vi "CRYGet detailed path information.vi"(11 "complete path":path) -> (2 "portion type":i16, 3 "longest valid portion":path)   [LabVIEW 2013]
panel:
  out "stripped?":bool
  # "0: empty\n1: directory\n2: existing file\n3: valid new file\n4: Not a Path"
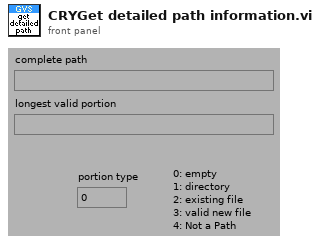
[diagram p1: front panel]
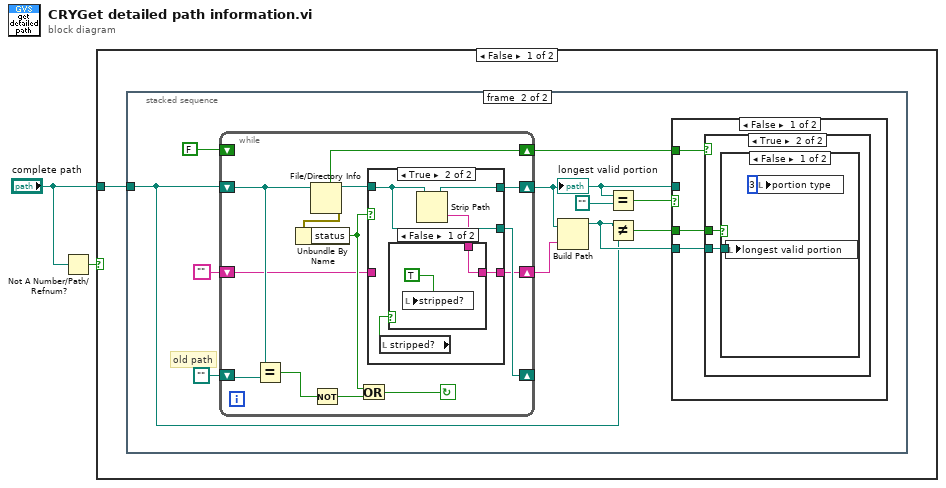
[diagram p0: block diagram]
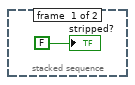
[diagram p2: hidden frame]
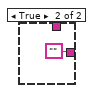
[diagram p4: hidden frame]
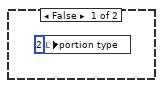
[diagram p5: hidden frame]
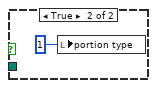
[diagram p6: hidden frame]
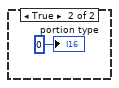
[diagram p7: hidden frame]
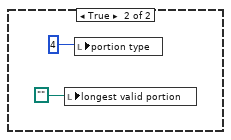
[diagram p8: hidden frame]
diagram:
  n1 = Not A Number/Path/Refnum?(number/path/refnum="complete path") -> (NaN/Path/Refnum?=w1:bool)
  n2 = case shown="False" w1 {
    tunnel: "complete path" -> [w3 _]
    frame False {
      n3 = stacked-sequence {
        tunnel: w3 -> [_ w5]
        frame #0 {
          "stripped?" <- FALSE
        }
        frame #1 {
          # "old path"
          n4 = while {
            shift-left: "" -> [w16]
            shift-right: [w17] -> w9
            shift-left: path "" -> [w22]
            shift-right: [w18] -> _
            shift-left: FALSE -> [_]
            shift-right: [w24] -> w11
            shift-left: w5 -> [w21]
            shift-right: [w23] -> w10
            stop <- w25 continue-if-true
            n5 = Equal?(x=w21, y=w22) -> (x = y?=w20:bool)
            n6 = File/Directory Info(path=w21) -> (path out=w27:path, directory=w24:bool, error out=w28:errorcluster)  [unwired: 1 in, 4 out]
            n7 = Unbundle By Name(w28) -> ("status"=w26:bool)
            n8 = Not(x=w20) -> (.not. x?=w19:bool)
            n9 = Or(x=w26, y=w19) -> (x .or. y?=w25:bool)
            n10 = case shown="True" w26 {
              tunnel: w27 -> [w30 w34]
              tunnel: [w30 w35] -> w23
              tunnel: [w30 w34] -> w18
              tunnel: [w29 w31] -> w17
              tunnel: w16 -> [w29 _]
              frame False {
              }
              frame True {
                n11 = local read "stripped?"() -> (w33:bool)
                n12 = Strip Path(path=w34) -> (stripped path=w35:path, name=w32:string)
                n13 = case shown="False" w33 {
                  tunnel: w32 -> [w37 _]
                  tunnel: [w37 ""] -> w31
                  frame False {
                    n14 = local write "stripped?"(TRUE ("stripped?")) -> ()
                  }
                  frame True {
                  }
                }
              }
            }
          }
          "longest valid portion" <- w10
          n15 = Build Path(base path=w10, name or relative path=w9) -> (appended path=w6:path)
          n16 = Equal?(x=w10, y=path "") -> (x = y?=w8:bool)
          n17 = Not Equal?(x=w6, y=w5) -> (x != y?=w7:bool)
          n18 = case shown="False" w8 {
            tunnel: w11 -> [w41 _]
            tunnel: w10 -> [_ _]
            tunnel: w7 -> [w40 _]
            tunnel: w6 -> [w39 _]
            frame False {
              n19 = case shown="True" w41 {
                tunnel: w40 -> [_ w44]
                tunnel: w39 -> [_ w43]
                frame False {
                  n20 = local write "portion type"(i16 2 ("portion type")) -> ()
                }
                frame True {
                  n21 = case shown="False" w44 {
                    tunnel: w43 -> [w45 _]
                    frame False {
                      n22 = local write "longest valid portion"(w45) -> ()
                      n23 = local write "portion type"(i16 3 ("portion type")) -> ()
                    }
                    frame True {
                      n24 = local write "portion type"(i16 1 ("portion type")) -> ()
                    }
                  }
                }
              }
            }
            frame True {
              "portion type" <- i16 0 ("portion type")
            }
          }
        }
      }
    }
    frame True {
      n25 = local write "longest valid portion"(path "") -> ()
      n26 = local write "portion type"(4) -> ()
    }
  }
